vi "Save Image.vi"(8 "error in (no error)":errorcluster, 11 "HIJ Vision Application in":refnum<class "HIJ Vision Application.lvclass">) -> (0 "error out":errorcluster, 3 "HIJ Vision Application out":refnum<class "HIJ Vision Application.lvclass">)   [LabVIEW 2014, in "HIJ Vision Application.lvlib" / "HIJ Vision Application.lvclass"]
uses:
  HIJ Vision Application.lvclass
  HIJ Vision Application.lvclass/HIJ Vision Application.ctl
  <vilib>/ActorFramework/Message Enqueuer/Message Enqueuer.lvclass/Message Enqueuer.ctl
  Read Display Enq.vi
  <vilib>/ActorFramework/Message Enqueuer/Enqueue.vi
  <vilib>/ActorFramework/Message Priority Queue/Priority Enqueue.vi
  <vilib>/ActorFramework/Message Enqueuer/Message Enqueuer.lvclass
  Display Actors/HIJ Vision Display/HIJ Vision Display Messages/Save Image Msg/Save Image Msg.lvclass
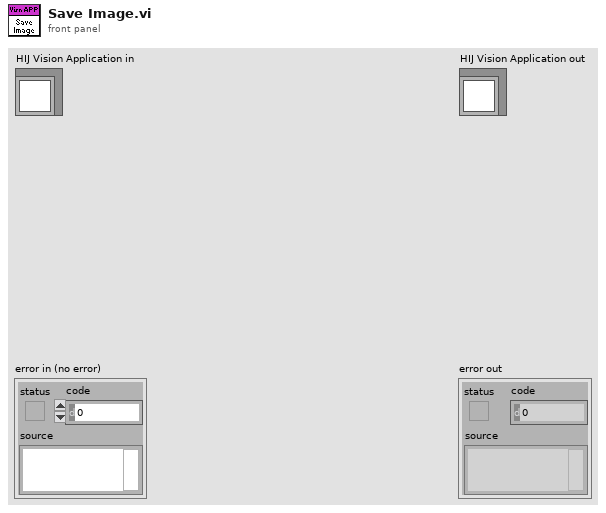
[diagram p1: front panel]
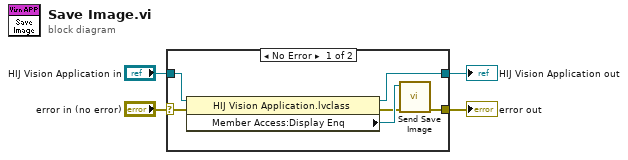
[diagram p0: block diagram]
diagram:
  n1 = case shown="No Error" "error in (no error)" {
    selector: "error in (no error)" -> [w8 w12]
    tunnel: [w5 w12] -> w3
    tunnel: [w9 w11] -> w1
    tunnel: "HIJ Vision Application in" -> [w10 w11]
    frame No Error {
      n2 = property class="HIJ Vision Application.lvclass"(reference=w10, error in=w8) -> (reference out=w9:refnum<class "HIJ Vision Application.lvclass">, error out=w6:errorcluster, "Member Access:Display Enq"=w7:refnum<class "Message Enqueuer.lvclass">)
      n3 = call "Send Save Image.vi"("error in (no error)"=w6, "Message Enqueuer"=w7) -> ("error out"=w5:errorcluster)  [unwired: 8 in, 1 out]
    }
    frame Error {
    }
  }
  "error out" <- w3
  "HIJ Vision Application out" <- w1
